vi "Teleop.vi"(10 "Match Info":T1={"Autonomous Elapsed Seconds"=0.0, "TeleOp Elapsed Seconds"=0.0, "Disabled Elapsed Seconds"=0.0, "Visited Autonomous"=FALSE, "Visited TeleOp"=FALSE, "Visited Disabled"=FALSE, "Autonomous Settings"={"Autonomous Style"=enum."Independent", "VI Refnum"=refnum}}, 11 "Call Context":T2) -> ()   [LabVIEW 2012]
doc: "This VI is called for each TeleOp packet received from the DS where the robot is not disabled. It is often used to read from the joysticks and update I/O or to update setpoints for timed control loops. It should complete and return within 20 milliseconds or it may miss DS packets."
uses:
  <vilib>/Rock Robotics/WPI/DriverStation/WPI_DriverStationDerivedRobotMode.ctl
  <vilib>/Rock Robotics/WPI/DriverStation/WPI_DriverStationMatch Info.ctl
  <vilib>/Rock Robotics/WPI/Relay/WPI_RelayValue.ctl
  Robot Global Data.vi
  <vilib>/Rock Robotics/WPI/Joystick/WPI_JoystickGetSetRefNum.vi
panel:
  out "Numeric 1":dbl(slide) scale=0.0..100.0
  out "Boolean 2":bool
  out "Boolean 1":bool
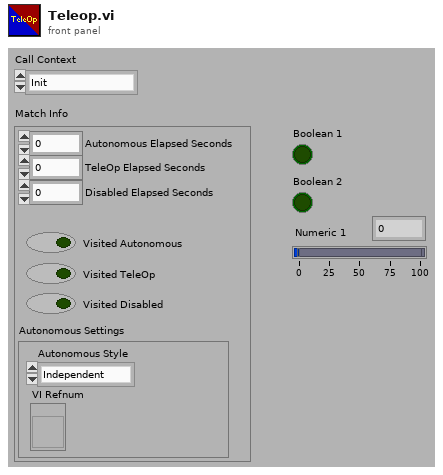
[diagram p1: front panel]
types:
  T1 = typedef "WPI_DriverStationMatch Info.ctl" = cluster{"Autonomous Elapsed Seconds":dbl, "TeleOp Elapsed Seconds":dbl, "Disabled Elapsed Seconds":dbl, "Visited Autonomous":bool, "Visited TeleOp":bool, "Visited Disabled":bool, "Autonomous Settings":cluster{"Autonomous Style":enum16{"Iterative", "Independent"}, "VI Refnum":refnum<vi>}}
  T2 = typedef "WPI_DriverStationDerivedRobotMode.ctl" = enum16{"Init", "Execute", "Stop"}
  T3 = typedef "WPI_RelayValue.ctl" = enum16{"Off", "On", "Forward", "Reverse"}
  T4 = typedef "WPI_JoystickDevRef.ctl" = cluster{"Device":T5}
  T5 = typedef "WPI_JoystickDeviceEnum.ctl" = enum16{"USB 1", "USB 2", "USB 3", "USB 4", "Kinect 1", "Kinect 2"}
  T6 = typedef "WPI_JoystickButtonState.ctl" = cluster{"Button 1":bool, "Button 2":bool, "Button 3":bool, "Button 4":bool, "Button 5":bool, "Button 6":bool, "Button 7":bool, "Button 8":bool, "Button 9":bool, "Button 10":bool, "Button 11":bool, "Button 12":bool}
  T7 = cluster{"axis 1 (x)":dbl, "axis 2 (y)":dbl, "axis 3 (throttle)":dbl, "axis 4":dbl, "axis 5":dbl, "axis 6":dbl}
  T8 = typedef "WPI_MotorControlDeviceRef.ctl" = cluster{"DeviceStatus":errorcluster, "Type":enum16{"PWM", "CAN"}, "PWM":cluster{"Digital Module":T9, "PWM Channel":T10, "DeadBand":T11}, "CAN":cluster{"Device Number":u8, "Control Mode":T12, "Semaphore":T13, "Max Vout":dbl}, "Invert":bool, "TransformRef":T14, "InvTransformRef":T14}
  T9 = typedef "FPGA_TypedefDigitalModule.ctl" = enum16{"Digital Module 1", "Digital Module 2"}
  T10 = typedef "FPGA_DIOPWMChannel.ctl" = enum8{"PWM 1", "PWM 2", "PWM 3", "PWM 4", "PWM 5", "PWM 6", "PWM 7", "PWM 8", "PWM 9", "PWM 10", "Invalid"}
  T11 = typedef "WPI_PWMDeadband.ctl" = cluster{"Name":string, "maxPositivePwm":i32, "minPositivePwm":i32, "centerPwm":i32, "maxNegativePwm":i32, "minNegativePwm":i32, "angularRange":u16}
  T12 = typedef "WPI_CANJaguar_ControlMode.ctl" = enum8{"Percent VBus", "Current", "Speed", "Position", "Voltage"}
  T13 = typedef "Semaphore RefNum" = refnum<k1>
  T14 = typedef "WPI_PWMTransform_ConPane.ctl" = refnum<vi>
  T15 = typedef "WPI_RelayDevRef.ctl" = cluster{"DevStatus":errorcluster, "Relay Channel":T16, "Digital Module":T9, "Relay Direction":T17}
  T16 = typedef "FPGA_DIORelayChannel.ctl" = enum8{"Relay 1", "Relay 2", "Relay 3", "Relay 4", "Relay 5", "Relay 6", "Relay 7", "Relay 8", "Invalid"}
  T17 = typedef "WPI_RelayDirection.ctl" = enum16{"Both directions", "Forward only", "Reverse only"}
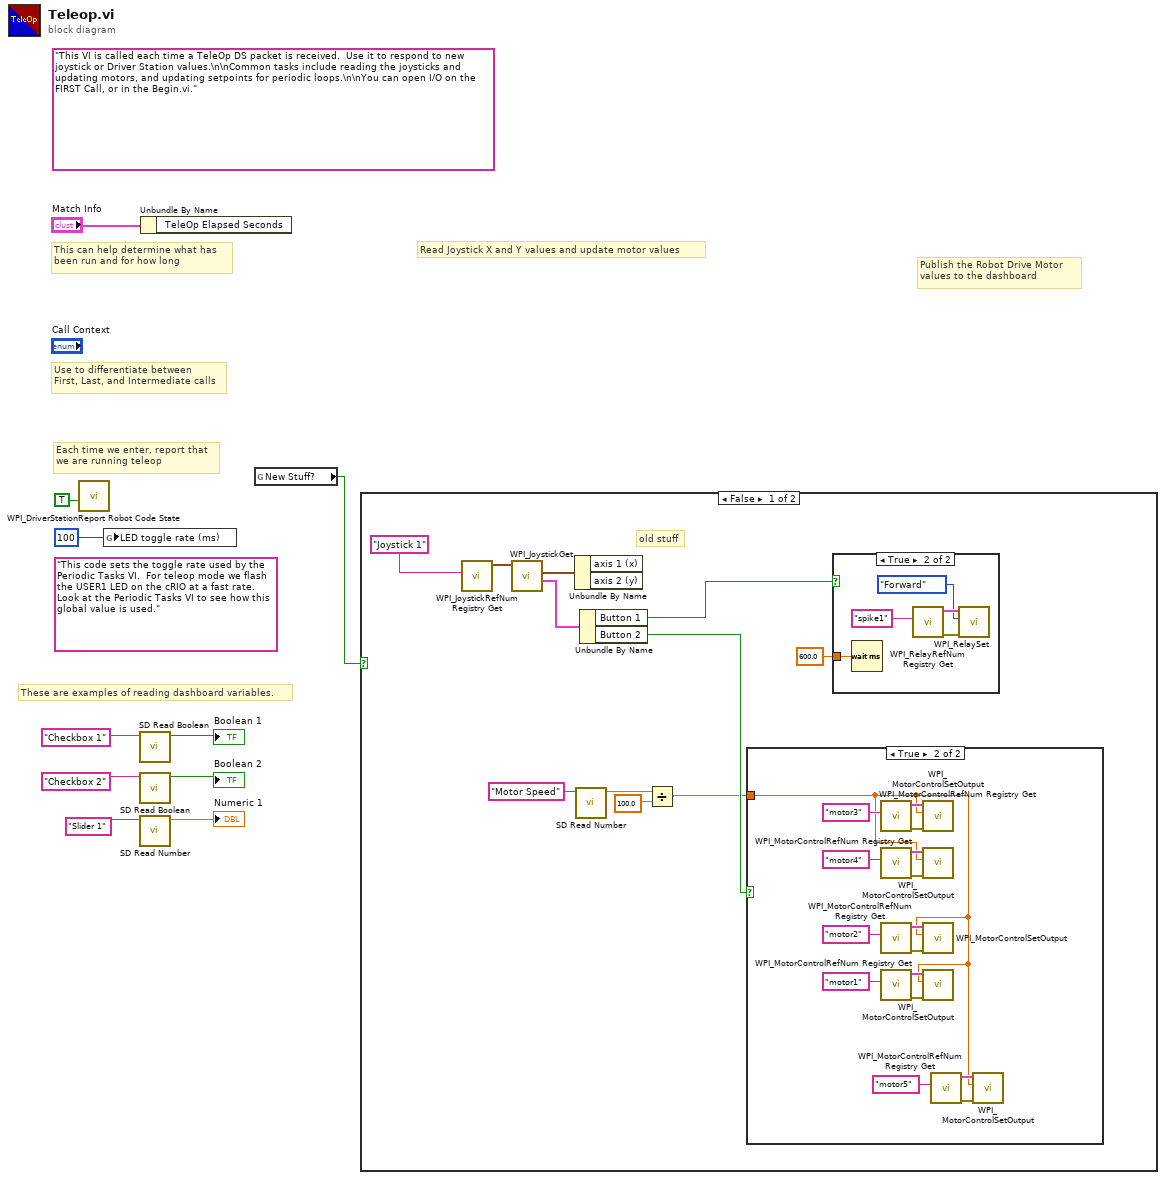
[diagram p0: block diagram]
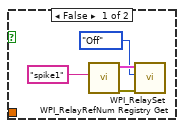
[diagram p2: hidden frame]
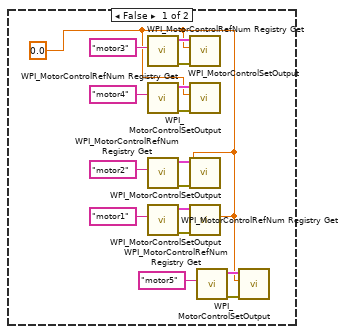
[diagram p3: hidden frame]
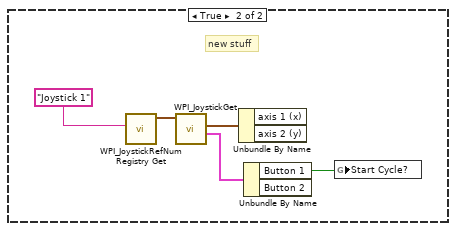
[diagram p4: hidden frame]
diagram:
  (unwired) "This code sets the toggle rate used by the Periodic Tasks VI.  For teleop mode we flash the USER1 LED on the cRIO at a fast rate.  Look at the Periodic Tasks VI to see how this global value is used."
  (unwired) "This VI is called each time a TeleOp DS packet is received.  Use it to respond to new joystick or Driver Station values.\n\nCommon tasks include reading the joysticks and updating motors, and updating setpoints for periodic loops.\n\nYou can open I/O on the FIRST Call, or in the Begin.vi."
  # "These are examples of reading dashboard variables."
  # "Publish the Robot Drive Motor\nvalues to the dashboard"
  # "Each time we enter, report that\nwe are running teleop"
  # "Use to differentiate between\nFirst, Last, and Intermediate calls"
  # "This can help determine what has\nbeen run and for how long"
  # "Read Joystick X and Y values and update motor values"
  n1 = call <vilib>:"WPI_DriverStationReport Robot Code State.vi"("TeleOp"=TRUE ("Autonomous")) -> ()  [unwired: 10 in, 1 out]
  n2 = global write "Robot Global Data.vi" "LED toggle rate (ms)"(u32 100 ("LED ms toggle rate")) -> ()
  n3 = call <vilib>:"SD Read Boolean.vi"("Name"="Checkbox 1" ("refnum name")) -> ("Boolean"=→"Boolean 1":bool)  [unwired: 8 in, 2 out]
  n4 = call <vilib>:"SD Read Boolean.vi"("Name"="Checkbox 2" ("refnum name")) -> ("Boolean"=→"Boolean 2":bool)  [unwired: 8 in, 2 out]
  n5 = call <vilib>:"SD Read Number.vi"("Name"="Slider 1" ("refnum name")) -> ("Numeric"=→"Numeric 1":dbl)  [unwired: 8 in, 2 out]
  n6 = Unbundle By Name("Match Info") -> ()  [unwired: 1 out]
  n7 = global read "Robot Global Data.vi" "New Stuff?"() -> (w1:bool)
  n8 = case shown="False" w1 {
    frame False {
      # "old stuff"
      n9 = call <vilib>:"WPI_JoystickRefNum Registry Get.vi"("refnum name"="Joystick 1") -> ("JoystickDevRef"=w20:T4)  [unwired: 1 in, 9 out]
      n10 = call <vilib>:"WPI_JoystickGet.vi"("JoystickDevRef"=w20) -> ("Buttons"=w18:T6, "Axes"=w19:T7)  [unwired: 1 in, 4 out]
      n11 = Unbundle By Name(w19) -> ()  [unwired: 2 out]
      n12 = call <vilib>:"SD Read Number.vi"("Name"="Motor Speed" ("refnum name")) -> ("Numeric"=w16:dbl)  [unwired: 8 in, 2 out]
      n13 = Unbundle By Name(w18) -> ("Button 1"=w12:bool, "Button 2"=w14:bool)
      n14 = Divide(x=w16, y=100.0) -> (x/y=w13:dbl)
      n15 = case shown="True" w14 {
        tunnel: w13 -> [_ w47]
        frame False {
          w31 = 0.0 ("Output")
          n16 = call <vilib>:"WPI_MotorControlRefNum Registry Get.vi"("refnum name"="motor3") -> ("error out"=w39:errorcluster, "MotorControlDevRef"=w40:T8)  [unwired: 9 in]
          n17 = call <vilib>:"WPI_MotorControlRefNum Registry Get.vi"("refnum name"="motor4") -> ("error out"=w36:errorcluster, "MotorControlDevRef"=w37:T8)  [unwired: 9 in]
          n18 = call <vilib>:"WPI_MotorControlRefNum Registry Get.vi"("refnum name"="motor2") -> ("error out"=w42:errorcluster, "MotorControlDevRef"=w43:T8)  [unwired: 9 in]
          n19 = call <vilib>:"WPI_MotorControlRefNum Registry Get.vi"("refnum name"="motor1") -> ("error out"=w45:errorcluster, "MotorControlDevRef"=w46:T8)  [unwired: 9 in]
          n20 = call <vilib>:"WPI_MotorControlSetOutput.vi"("error in (no error)"=w39, "Output"=w31, "MotorControlDevRef"=w40) -> ()  [unwired: 6 in, 3 out]
          n21 = call <vilib>:"WPI_MotorControlSetOutput.vi"("error in (no error)"=w36, "Output"=w31, "MotorControlDevRef"=w37) -> ()  [unwired: 6 in, 3 out]
          n22 = call <vilib>:"WPI_MotorControlSetOutput.vi"("error in (no error)"=w42, "Output"=w31, "MotorControlDevRef"=w43) -> ()  [unwired: 6 in, 3 out]
          n23 = call <vilib>:"WPI_MotorControlSetOutput.vi"("error in (no error)"=w45, "Output"=w31, "MotorControlDevRef"=w46) -> ()  [unwired: 6 in, 3 out]
          n24 = call <vilib>:"WPI_MotorControlRefNum Registry Get.vi"("refnum name"="motor5") -> ("error out"=w33:errorcluster, "MotorControlDevRef"=w34:T8)  [unwired: 9 in]
          n25 = call <vilib>:"WPI_MotorControlSetOutput.vi"("error in (no error)"=w33, "Output"=w31, "MotorControlDevRef"=w34) -> ()  [unwired: 6 in, 3 out]
        }
        frame True {
          n26 = call <vilib>:"WPI_MotorControlRefNum Registry Get.vi"("refnum name"="motor3") -> ("error out"=w55:errorcluster, "MotorControlDevRef"=w56:T8)  [unwired: 9 in]
          n27 = call <vilib>:"WPI_MotorControlRefNum Registry Get.vi"("refnum name"="motor4") -> ("error out"=w52:errorcluster, "MotorControlDevRef"=w53:T8)  [unwired: 9 in]
          n28 = call <vilib>:"WPI_MotorControlRefNum Registry Get.vi"("refnum name"="motor2") -> ("error out"=w58:errorcluster, "MotorControlDevRef"=w59:T8)  [unwired: 9 in]
          n29 = call <vilib>:"WPI_MotorControlRefNum Registry Get.vi"("refnum name"="motor1") -> ("error out"=w61:errorcluster, "MotorControlDevRef"=w62:T8)  [unwired: 9 in]
          n30 = call <vilib>:"WPI_MotorControlSetOutput.vi"("error in (no error)"=w55, "Output"=w47, "MotorControlDevRef"=w56) -> ()  [unwired: 6 in, 3 out]
          n31 = call <vilib>:"WPI_MotorControlSetOutput.vi"("error in (no error)"=w52, "Output"=w47, "MotorControlDevRef"=w53) -> ()  [unwired: 6 in, 3 out]
          n32 = call <vilib>:"WPI_MotorControlSetOutput.vi"("error in (no error)"=w58, "Output"=w47, "MotorControlDevRef"=w59) -> ()  [unwired: 6 in, 3 out]
          n33 = call <vilib>:"WPI_MotorControlSetOutput.vi"("error in (no error)"=w61, "Output"=w47, "MotorControlDevRef"=w62) -> ()  [unwired: 6 in, 3 out]
          n34 = call <vilib>:"WPI_MotorControlRefNum Registry Get.vi"("refnum name"="motor5") -> ("error out"=w49:errorcluster, "MotorControlDevRef"=w50:T8)  [unwired: 9 in]
          n35 = call <vilib>:"WPI_MotorControlSetOutput.vi"("error in (no error)"=w49, "Output"=w47, "MotorControlDevRef"=w50) -> ()  [unwired: 6 in, 3 out]
        }
      }
      n36 = case shown="True" w12 {
        tunnel: 600.0 ("Timed Cycle") -> [_ w30]
        frame False {
          n37 = call <vilib>:"WPI_RelayRefNum Registry Get.vi"("refnum name"="spike1") -> ("error out"=w25:errorcluster, "RelayDevRef"=w24:T15)  [unwired: 9 in]
          n38 = call <vilib>:"WPI_RelaySet.vi"("error in (no error)"=w25, "RelayValue"=WPI_RelayValue."Off", "RelayDevRef"=w24) -> ()  [unwired: 7 in, 2 out]
        }
        frame True {
          n39 = Wait (ms)(milliseconds to wait=w30) -> ()  [unwired: 1 out]
          n40 = call <vilib>:"WPI_RelayRefNum Registry Get.vi"("refnum name"="spike1") -> ("error out"=w29:errorcluster, "RelayDevRef"=w28:T15)  [unwired: 9 in]
          n41 = call <vilib>:"WPI_RelaySet.vi"("error in (no error)"=w29, "RelayValue"=WPI_RelayValue."Forward", "RelayDevRef"=w28) -> ()  [unwired: 7 in, 2 out]
        }
      }
    }
    frame True {
      # "new stuff"
      n42 = call <vilib>:"WPI_JoystickRefNum Registry Get.vi"("refnum name"="Joystick 1") -> ("JoystickDevRef"=w66:T4)  [unwired: 1 in, 9 out]
      n43 = call <vilib>:"WPI_JoystickGet.vi"("JoystickDevRef"=w66) -> ("Buttons"=w64:T6, "Axes"=w65:T7)  [unwired: 1 in, 4 out]
      n44 = Unbundle By Name(w65) -> ()  [unwired: 2 out]
      n45 = Unbundle By Name(w64) -> ("Button 1"=w63:bool)  [unwired: 1 out]
      n46 = global write "Robot Global Data.vi" "Start Cycle?"(w63) -> ()
    }
  }
